vi "GetManualCommands.vi"(11 "Manual Script Entry (0)":string) -> (3 "Commands":string[](array[string]))   [LabVIEW 2018]
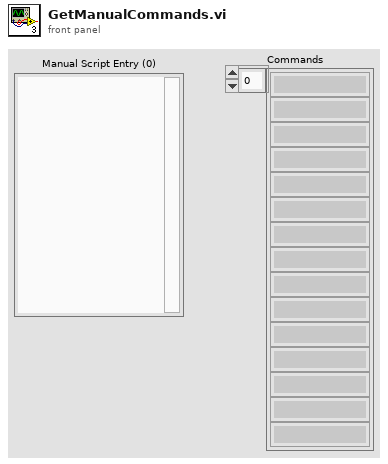
[diagram p1: front panel]
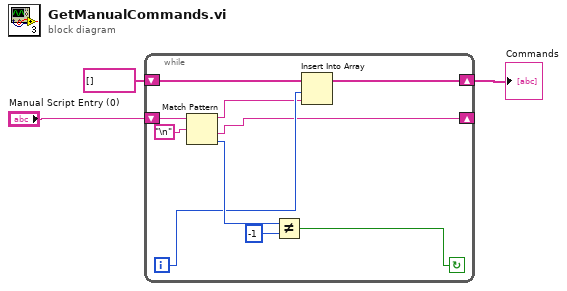
[diagram p0: block diagram]
diagram:
  n1 = while {
    shift-right: [w6] -> _
    shift-left: "Manual Script Entry (0)" -> [w13]
    shift-right: [w5] -> w1
    shift-left: string[] [] -> [w4]
    i -> [w8]
    stop <- w10 continue-if-true
    n2 = Match Pattern(string=w13, regular expression="\n") -> (before substring=w7:string, after substring=w6:string, offset past match=w12:i32)  [unwired: 1 in, 1 out]
    n3 = Not Equal?(x=w12, y=-1) -> (x != y?=w10:bool)
    n4 = Insert Into Array(array=w4, index=w8, new element=w7) -> (w5:string[])
  }
  "Commands" <- w1
